vi "iWorx 2 pt Scale.vi"(7 "Set Points":T1={"SP1 Voltage"=1.0, "SP1 Value"=5.0, "SP2 Voltage"=1.0, "SP2 Value"=5.0} {"SP2 Value" format="%.1f mS"; "SP2 Voltage" format="%.1f V"; "SP1 Value" format="%.1f mS"; "SP1 Voltage" format="%.1f V"}, 9 "Offset in":dbl=nan, 10 "Slope in":dbl=nan, 11 "Raw Waveform":waveform(dbl)) -> (1 "Offset":dbl, 2 "Slope":dbl, 3 "Scaled Value":waveform(dbl))   [LabVIEW 2012]
doc: "This subVI takes a waveform input and will apply a linear scale (Y=mx+b) based on two (X,Y) Set Points.\nIf you input a specific <b>slope</b> and <b> offset</b> it will override the set point and apply the desired scaling."
uses:
  iWorx Set Points.ctl
panel:
  # "(              ,              )"
  # "(              ,              )"
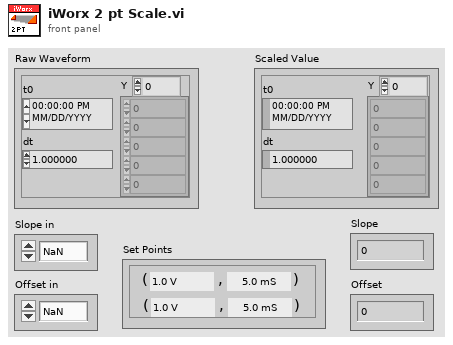
[diagram p1: front panel]
types:
  T1 = typedef "iWorx Set Points.ctl" = cluster{"SP1 Voltage":dbl, "SP1 Value":dbl, "SP2 Voltage":dbl, "SP2 Value":dbl}
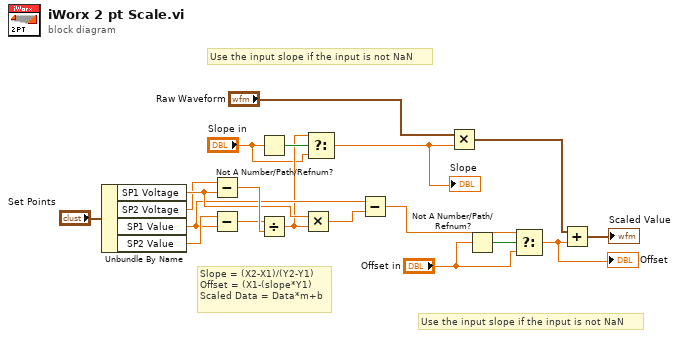
[diagram p0: block diagram]
diagram:
  # "Use the input slope if the input is not NaN"
  # "Use the input slope if the input is not NaN"
  # "Slope = (X2-X1)/(Y2-Y1)\nOffset = (X1-(slope*Y1)\nScaled Data = Data*m+b"
  n1 = Unbundle By Name("Set Points") -> ("SP1 Voltage"=w14:dbl, "SP2 Voltage"=w13:dbl, "SP1 Value"=w11:dbl, "SP2 Value"=w12:dbl)
  n2 = Subtract(x=w13, y=w14) -> (x-y=w17:dbl)
  n3 = Subtract(x=w12, y=w11) -> (x-y=w16:dbl)
  n4 = Not A Number/Path/Refnum?(number/path/refnum="Slope in") -> (NaN/Path/Refnum?=w10:bool)
  n5 = Divide(x=w16, y=w17) -> (x/y=w9:dbl)
  n6 = Multiply(x=w14, y=w9) -> (x*y=w18:dbl)
  n7 = Select(t=w9, s=w10, f="Slope in") -> (s? t:f=w7:dbl)
  "Slope" <- w7
  n8 = Subtract(x=w11, y=w18) -> (x-y=w6:dbl)
  n9 = Multiply(x="Raw Waveform", y=w7) -> (x*y=w19:waveform(dbl))
  n10 = Not A Number/Path/Refnum?(number/path/refnum="Offset in") -> (NaN/Path/Refnum?=w4:bool)
  n11 = Select(t=w6, s=w4, f="Offset in") -> (s? t:f=w3:dbl)
  "Offset" <- w3
  n12 = Add(x=w19, y=w3) -> (x+y=→"Scaled Value":waveform(dbl))
